vi "CheckSpectrumSFAT.vi"(8 "error in":errorcluster, 10 "SFAT Settings":T1, 11 "connection ID in":refnum<k5>) -> (0 "error out":errorcluster, 1 "Error Info":T3, 2 "OK":bool, 3 "connection ID out":refnum<k5>, 4 "Log String":string, 5 "Checked Spectrum Parameters":T2 {"Step Width" format="%#.3g"})   [LabVIEW 2020, in "ProdigyRemoteControl.lvlib"]
uses:
  ProdigyRemoteControl.lvlib
  DEFINITIONS/DEF_RcError.ctl
  DEFINITIONS/DEF_ValSpectrParas.ctl
  DEFINITIONS/DEF_SFAT_Settings.ctl
  DEFINITIONS/DEF_RcCmd.ctl
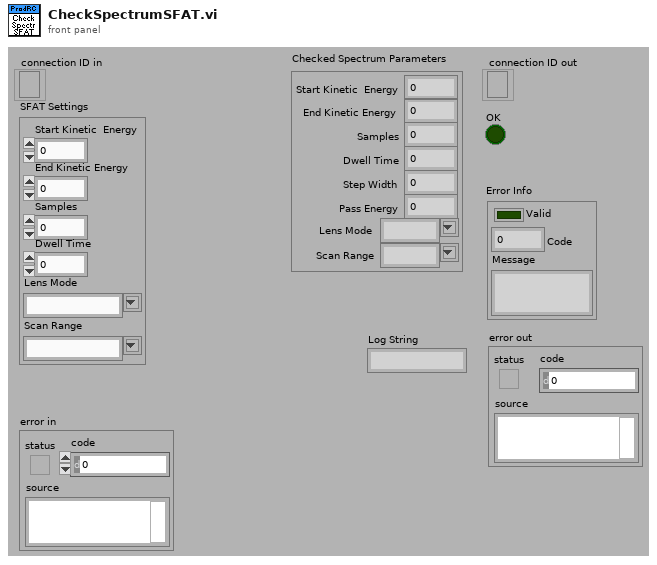
[diagram p1: front panel]
types:
  T1 = typedef "ProdigyRemoteControl.lvlib/DEF_SFAT_Settings.ctl" = cluster{"Start Kinetic  Energy":dbl, "End Kinetic Energy":dbl, "Samples":u32, "Dwell Time":dbl, "Scan Range":string, "Lens Mode":string}
  T2 = typedef "ProdigyRemoteControl.lvlib/DEF_ValSpectrParas.ctl" = cluster{"Start Kinetic  Energy":dbl, "End Kinetic Energy":dbl, "Samples":u32, "Dwell Time":dbl, "Step Width":dbl, "Pass Energy":dbl, "Lens Mode":string, "Scan Range":string}
  T3 = typedef "ProdigyRemoteControl.lvlib/DEF_RcError.ctl" = cluster{"Valid":bool, "Code":u16, "Message":string}
  T4 = typedef "ProdigyRemoteControl.lvlib/DEF_RcCmd.ctl" = string
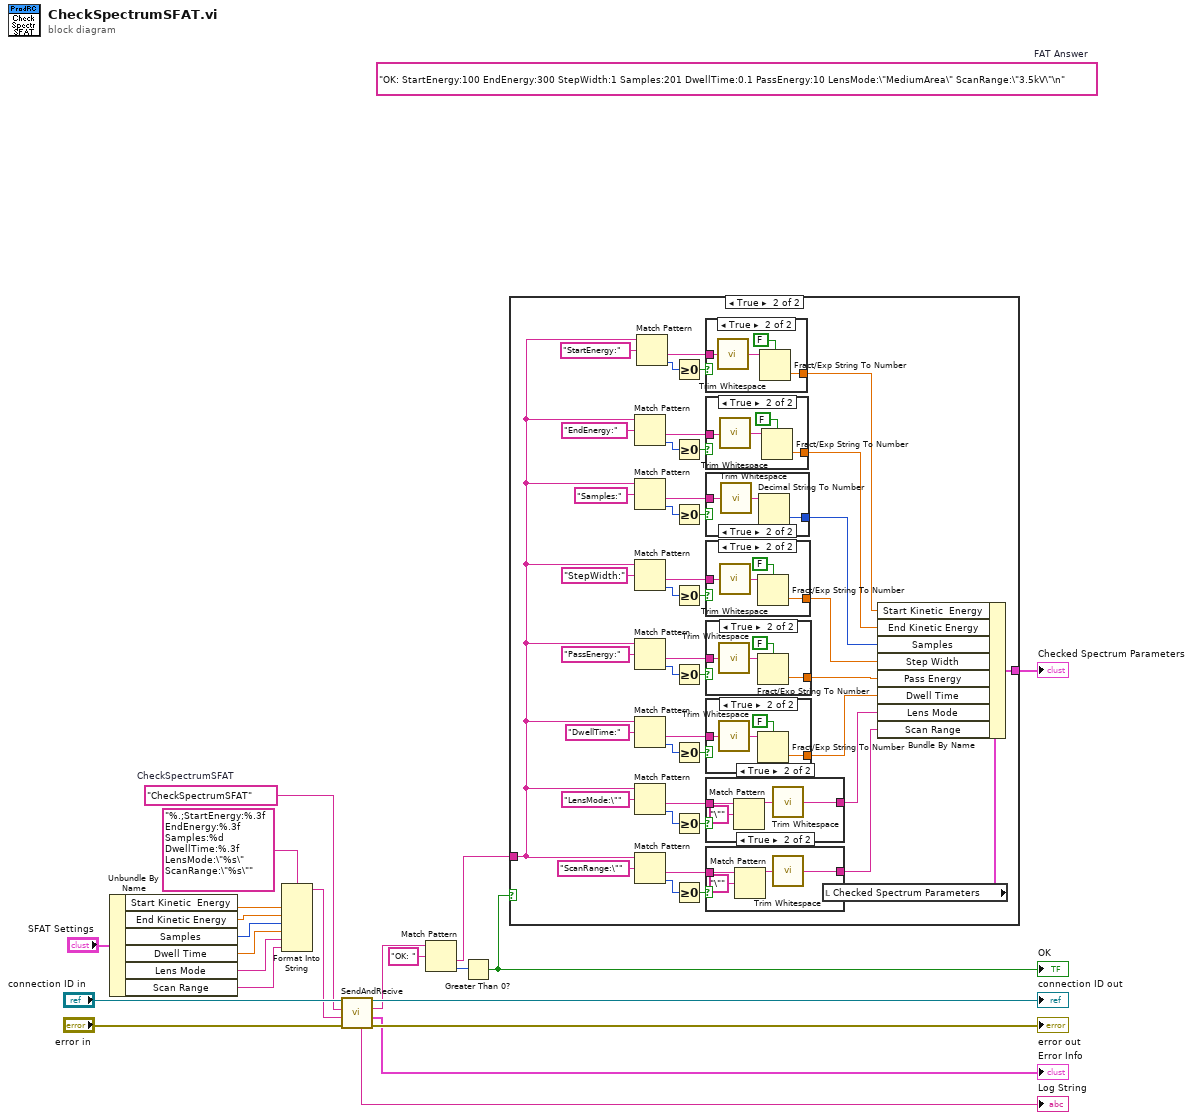
[diagram p0: block diagram]
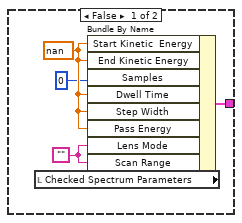
[diagram p2: hidden frame]
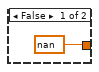
[diagram p3: hidden frame]
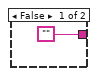
[diagram p4: hidden frame]
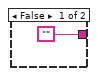
[diagram p5: hidden frame]
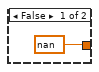
[diagram p6: hidden frame]
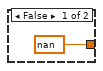
[diagram p7: hidden frame]
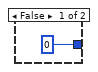
[diagram p8: hidden frame]
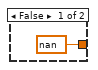
[diagram p9: hidden frame]
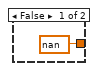
[diagram p10: hidden frame]
diagram:
  (unwired) "OK: StartEnergy:100 EndEnergy:300 StepWidth:1 Samples:201 DwellTime:0.1 PassEnergy:10 LensMode:\"MediumArea\" ScanRange:\"3.5kV\"\n"  # FAT Answer
  w10 = T4 "CheckSpectrumSFAT"  # CheckSpectrumSFAT
  n1 = Unbundle By Name("SFAT Settings") -> ("Start Kinetic  Energy"=w9:dbl, "End Kinetic Energy"=w8:dbl, "Samples"=w7:u32, "Dwell Time"=w6:dbl, "Lens Mode"=w5:string, "Scan Range"=w4:string)
  n2 = Format Into String(format string="%.;StartEnergy:%.3f EndEnergy:%.3f Samples:%d DwellTime:%.3f LensMode:\"%s\" ScanRange:\"%s\"", w9, w8, w7, w6, w5, w4) -> (resulting string=w2:string)  [unwired: 2 in, 1 out]
  n3 = call "SendAndRecive.vi"("error in"="error in", "Parameters"=w2, "Command"=w10, "connection ID in"="connection ID in") -> ("error out"=→"error out":errorcluster, "Error Info"=→"Error Info":T3, "Answer"=w16:string, "connection ID out"=→"connection ID out":refnum<k5>, "Log String"=→"Log String":string)  [unwired: 3 in]
  n4 = Match Pattern(string=w16, regular expression="OK: ") -> (after substring=w12:string, offset past match=w14:i32)  [unwired: 1 in, 2 out]
  n5 = Greater Than 0?(x=w14) -> (x > 0?=w11:bool)
  "OK" <- w11
  n6 = case shown="True" w11 {
    tunnel: w12 -> [_ w28]
    tunnel: [w26 w56] -> w13
    frame False {
      w23 = ""
      w25 = nan ("Start Kinetic  Energy")
      n7 = local read "Checked Spectrum Parameters"() -> (w27:T2)
      n8 = Bundle By Name(cluster=w27, "Start Kinetic  Energy"=w25, "End Kinetic Energy"=w25, "Samples"=u32 0, "Dwell Time"=w25, "Step Width"=w25, "Pass Energy"=w25, "Lens Mode"=w23, "Scan Range"=w23) -> (w26:T2)
    }
    frame True {
      n9 = Match Pattern(string=w28, regular expression="EndEnergy:") -> (after substring=w64:string, offset past match=w63:i32)  [unwired: 1 in, 2 out]
      n10 = Match Pattern(string=w28, regular expression="Samples:") -> (after substring=w61:string, offset past match=w60:i32)  [unwired: 1 in, 2 out]
      n11 = Match Pattern(string=w28, regular expression="StepWidth:") -> (after substring=w58:string, offset past match=w59:i32)  [unwired: 1 in, 2 out]
      n12 = Match Pattern(string=w28, regular expression="PassEnergy:") -> (after substring=w53:string, offset past match=w54:i32)  [unwired: 1 in, 2 out]
      n13 = Match Pattern(string=w28, regular expression="DwellTime:") -> (after substring=w34:string, offset past match=w33:i32)  [unwired: 1 in, 2 out]
      n14 = Match Pattern(string=w28, regular expression="LensMode:\"") -> (after substring=w48:string, offset past match=w47:i32)  [unwired: 1 in, 2 out]
      n15 = Match Pattern(string=w28, regular expression="ScanRange:\"") -> (after substring=w45:string, offset past match=w46:i32)  [unwired: 1 in, 2 out]
      n16 = Match Pattern(string=w28, regular expression="StartEnergy:") -> (after substring=w67:string, offset past match=w69:i32)  [unwired: 1 in, 2 out]
      n17 = Greater Or Equal To 0?(x=w69) -> (x >= 0?=w68:bool)
      n18 = Greater Or Equal To 0?(x=w63) -> (x >= 0?=w66:bool)
      n19 = Greater Or Equal To 0?(x=w60) -> (x >= 0?=w62:bool)
      n20 = Greater Or Equal To 0?(x=w59) -> (x >= 0?=w57:bool)
      n21 = Greater Or Equal To 0?(x=w54) -> (x >= 0?=w51:bool)
      n22 = Greater Or Equal To 0?(x=w33) -> (x >= 0?=w35:bool)
      n23 = Greater Or Equal To 0?(x=w47) -> (x >= 0?=w50:bool)
      n24 = Greater Or Equal To 0?(x=w46) -> (x >= 0?=w43:bool)
      n25 = case shown="True" w68 {
        tunnel: w67 -> [_ w109]
        tunnel: [nan w107] -> w42
        frame False {
        }
        frame True {
          n26 = call <vilib>:"Trim Whitespace.vi"("string"=w109) -> ("trimmed string"=w108:string)  [unwired: 1 in]
          n27 = Fract/Exp String To Number(use system decimal point (T)=FALSE, string=w108) -> (number=w107:dbl)  [unwired: 2 in, 1 out]
        }
      }
      n28 = case shown="True" w66 {
        tunnel: w64 -> [_ w104]
        tunnel: [nan w101] -> w41
        frame False {
        }
        frame True {
          n29 = call <vilib>:"Trim Whitespace.vi"("string"=w104) -> ("trimmed string"=w103:string)  [unwired: 1 in]
          n30 = Fract/Exp String To Number(use system decimal point (T)=FALSE, string=w103) -> (number=w101:dbl)  [unwired: 2 in, 1 out]
        }
      }
      n31 = case shown="True" w62 {
        tunnel: w61 -> [_ w99]
        tunnel: [0 w97] -> w39
        frame False {
        }
        frame True {
          n32 = call <vilib>:"Trim Whitespace.vi"("string"=w99) -> ("trimmed string"=w98:string)  [unwired: 1 in]
          n33 = Decimal String To Number(string=w98) -> (number=w97:i32)  [unwired: 2 in, 1 out]
        }
      }
      n34 = case shown="True" w57 {
        tunnel: w58 -> [_ w95]
        tunnel: [nan w92] -> w37
        frame False {
        }
        frame True {
          n35 = call <vilib>:"Trim Whitespace.vi"("string"=w95) -> ("trimmed string"=w93:string)  [unwired: 1 in]
          n36 = Fract/Exp String To Number(use system decimal point (T)=FALSE, string=w93) -> (number=w92:dbl)  [unwired: 2 in, 1 out]
        }
      }
      n37 = case shown="True" w51 {
        tunnel: w53 -> [_ w90]
        tunnel: [nan w87] -> w36
        frame False {
        }
        frame True {
          n38 = call <vilib>:"Trim Whitespace.vi"("string"=w90) -> ("trimmed string"=w88:string)  [unwired: 1 in]
          n39 = Fract/Exp String To Number(use system decimal point (T)=FALSE, string=w88) -> (number=w87:dbl)  [unwired: 2 in, 1 out]
        }
      }
      n40 = case shown="True" w35 {
        tunnel: w34 -> [_ w75]
        tunnel: [nan w72] -> w31
        frame False {
        }
        frame True {
          n41 = call <vilib>:"Trim Whitespace.vi"("string"=w75) -> ("trimmed string"=w73:string)  [unwired: 1 in]
          n42 = Fract/Exp String To Number(use system decimal point (T)=FALSE, string=w73) -> (number=w72:dbl)  [unwired: 2 in, 1 out]
        }
      }
      n43 = case shown="True" w50 {
        tunnel: w48 -> [_ w85]
        tunnel: ["" w84] -> w30
        frame False {
        }
        frame True {
          n44 = Match Pattern(string=w85, regular expression="\"") -> (before substring=w83:string)  [unwired: 1 in, 3 out]
          n45 = call <vilib>:"Trim Whitespace.vi"("string"=w83) -> ("trimmed string"=w84:string)  [unwired: 1 in]
        }
      }
      n46 = case shown="True" w43 {
        tunnel: w45 -> [_ w80]
        tunnel: ["" w79] -> w29
        frame False {
        }
        frame True {
          n47 = Match Pattern(string=w80, regular expression="\"") -> (before substring=w78:string)  [unwired: 1 in, 3 out]
          n48 = call <vilib>:"Trim Whitespace.vi"("string"=w78) -> ("trimmed string"=w79:string)  [unwired: 1 in]
        }
      }
      n49 = local read "Checked Spectrum Parameters"() -> (w55:T2)
      n50 = Bundle By Name(cluster=w55, "Start Kinetic  Energy"=w42, "End Kinetic Energy"=w41, "Samples"=w39, "Step Width"=w37, "Pass Energy"=w36, "Dwell Time"=w31, "Lens Mode"=w30, "Scan Range"=w29) -> (w56:T2)
    }
  }
  "Checked Spectrum Parameters" <- w13
